vi "Check Message Queue Status.vi"(0 "message queue in":T1, 11 "error in":errorcluster) -> (2 "max queue size":i32, 3 "message queue name":string, 4 "message queue out":T1, 6 "# elements in queue":i32, 15 "error out":errorcluster)   [LabVIEW 2015, in "TLB` Template.lvlib" / "AMC.lvlib"]
doc: "Returns the max queue size, message queue name, and the number of elements in the queue.TLB Prime - Application Template 1.3.0.24\nNorm Kirchner, NI Systems Engineering - NI\nCopyright (c) 2014, NI"
uses:
  AMC.lvlib
  Message Queue.ctl
  Message.ctl
  Tools/Keyed Array/KeyedArray.ctl
  Tools/Keyed Array/Tools_KeyedArray.lvlib
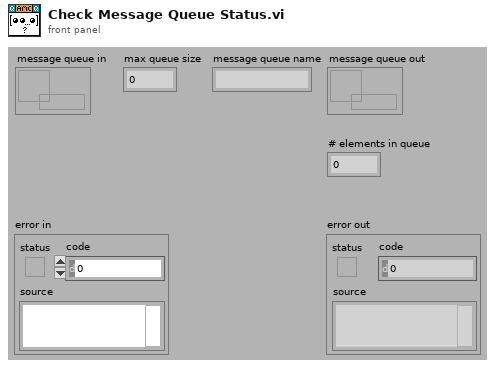
[diagram p1: front panel]
types:
  T1 = typedef "TLB` Template.lvlib/AMC.lvlib/Message Queue.ctl" = refnum<queue>
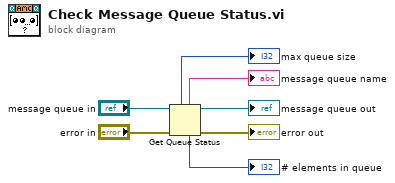
[diagram p0: block diagram]
diagram:
  n1 = Get Queue Status(queue="message queue in", error in (no error)="error in") -> (queue out=→"message queue out":T1, queue name=→"message queue name":string, max queue size=→"max queue size":i32, error out=→"error out":errorcluster, # elements in queue=→"# elements in queue":i32)  [unwired: 4 out]
